vi "StartSeveralKeihtley6221.vi"() -> ()   [LabVIEW 2025]
doc: "Author: Scott Hannahs <sth@magnet.fsu.edu>\n\nThis software is licensed for use under the “MIT License\"\nCopyright (c) 2025 Scott Hannahs, sth@sth@magnet.sthnet.net\n\nPermission is hereby granted, free of charge, to any person obtaining a copy of this software and associated documentation files (the \"Software\"), to deal in the Software without restriction, including without limitation the rights to use, copy, modify, merge, publish, distribute, sublicense, and/or sell copies of the Software, and to permit persons to whom the Software is furnished to do so, subject to the following conditions: The above copyright notice and this permission notice shall be included in all copies or substantial portions of the Software.\n\nTHE SOFTWARE IS PROVIDED \"AS IS\", WITHOUT WARRANTY OF ANY KIND, EXPRESS OR IMPLIED, INCLUDING BUT NOT LIMITED TO THE WARRANTIES OF MERCHANTABILITY, FITNESS FOR A PARTICULAR PURPOSE AND NONINFRINGEMENT. IN NO EVENT SHALL THE AUTHORS OR COPYRIGHT HOLDERS BE LIABLE FOR ANY CLAIM, DAMAGES OR OTHER LIABILITY, WHETHER IN AN ACTION OF CONTRACT, TORT OR OTHERWISE, ARISING FROM, OUT OF OR IN CONNECTION WITH THE SOFTWARE OR THE USE OR OTHER DEALINGS IN THE SOFTWARE."
panel:
  in  "stop":bool
  in  "RUN Button":bool
  in  "MODE":T1(tab)=enum."DELTA mode"
  in  "DELTA HIGH \n(0 --- +0.105 Amp)":dbl=5e-08 min=0.0 max=0.00105 format="%^.5e"
  in  "DELTA LOW \n(-0.105 --- 0 Amp)":dbl=-5e-08 min=-0.00105 max=0.0 format="%^.5e"
  in  "DELTA DELAY \n(0 --- 9999.999 sec)":dbl=0.1 min=0.0 max=9999.999 format="%^.5e"
  in  "Ilow = -Ihigh":bool=TRUE
  in  "Delay of 6221#d \nwith respect to 6221#s\n(sec)":dbl=0.01 min=0.0 max=9999.999 format="%^.5e"
  in  "apperture of 2181A#s \n(NPLC, integer 1 - 60)":dbl=1.0 min=0.0 max=9999.999 format="%^.5e"
  in  "Delay of 2182#d \nwith respect to 2182#s\n(NPLC, integer 1-59)\nType Zero, if serial connection":dbl min=0.0 max=9999.999 format="%^.5e"
  in  "DELAY \n(0 --- 9999.999 sec)":dbl=0.1 min=0.0 max=9999.999 format="%^.5e"
  in  "Time Delay of 6221#d \nwith respect to 6221#s \n(sec)":dbl=0.01 min=0.0 max=9999.999 format="%^.5e"
  in  "Apperture of 2182#s \n(NPLC, integer 1 - 60)":dbl=1.0 min=0.0 max=9999.999 format="%^.5e"
  in  "Delay of 2182#d \nwith respect to 2182#s\n(NPLC, integer 1-59)\nType Zero, if serial connection":dbl=1.0 min=0.0 max=9999.999 format="%^.5e"
  in  "DELTA == dI\n(0 --- +105 mA)":dbl=1e-08 min=0.0 max=0.00105 format="%^.5e"
  in  "STEP \n(0 --- +0.105 Amp)":dbl=2e-09 min=0.0 max=0.00105 format="%^.5e"
  in  "STOP \n(-105 -- +105 mA)":dbl=1e-06 min=-0.001 max=0.00105 format="%^.5e"
  in  "START\n(-105 -- +0.105 mA)":dbl=-1.2e-06 min=-0.001 max=0.00105 format="%^.5e"
  in  "Disable Displays":bool
  in  "Subordinate 6221s: Reinitialize to Default Value \nto reduce the amount of the elements":refnum<visa-resource-name>[](array[refnum])=["GPIB0::17::INSTR"]
  in  "Dominate Current source: 6221#d":refnum<visa-resource-name>="GPIB0::16::INSTR"
  # "Abort Sweep, Delta, Pulse Delta, or Differential Conductance immediately"
  # "Trigger armed mode. For example, Diff. conductance"
  # "1NPLC = 16.6[6]msec"
  # "1NPLC = 16.6[6]msec"
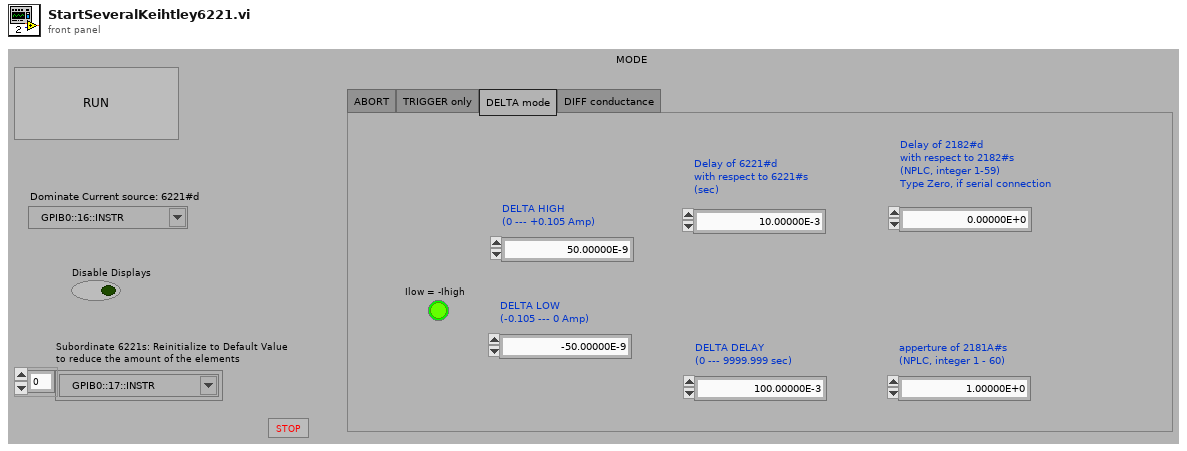
[diagram p1: front panel]
types:
  T1 = enum32{"ABORT", "TRIGGER only", "DELTA mode", "DIFF conductance"}
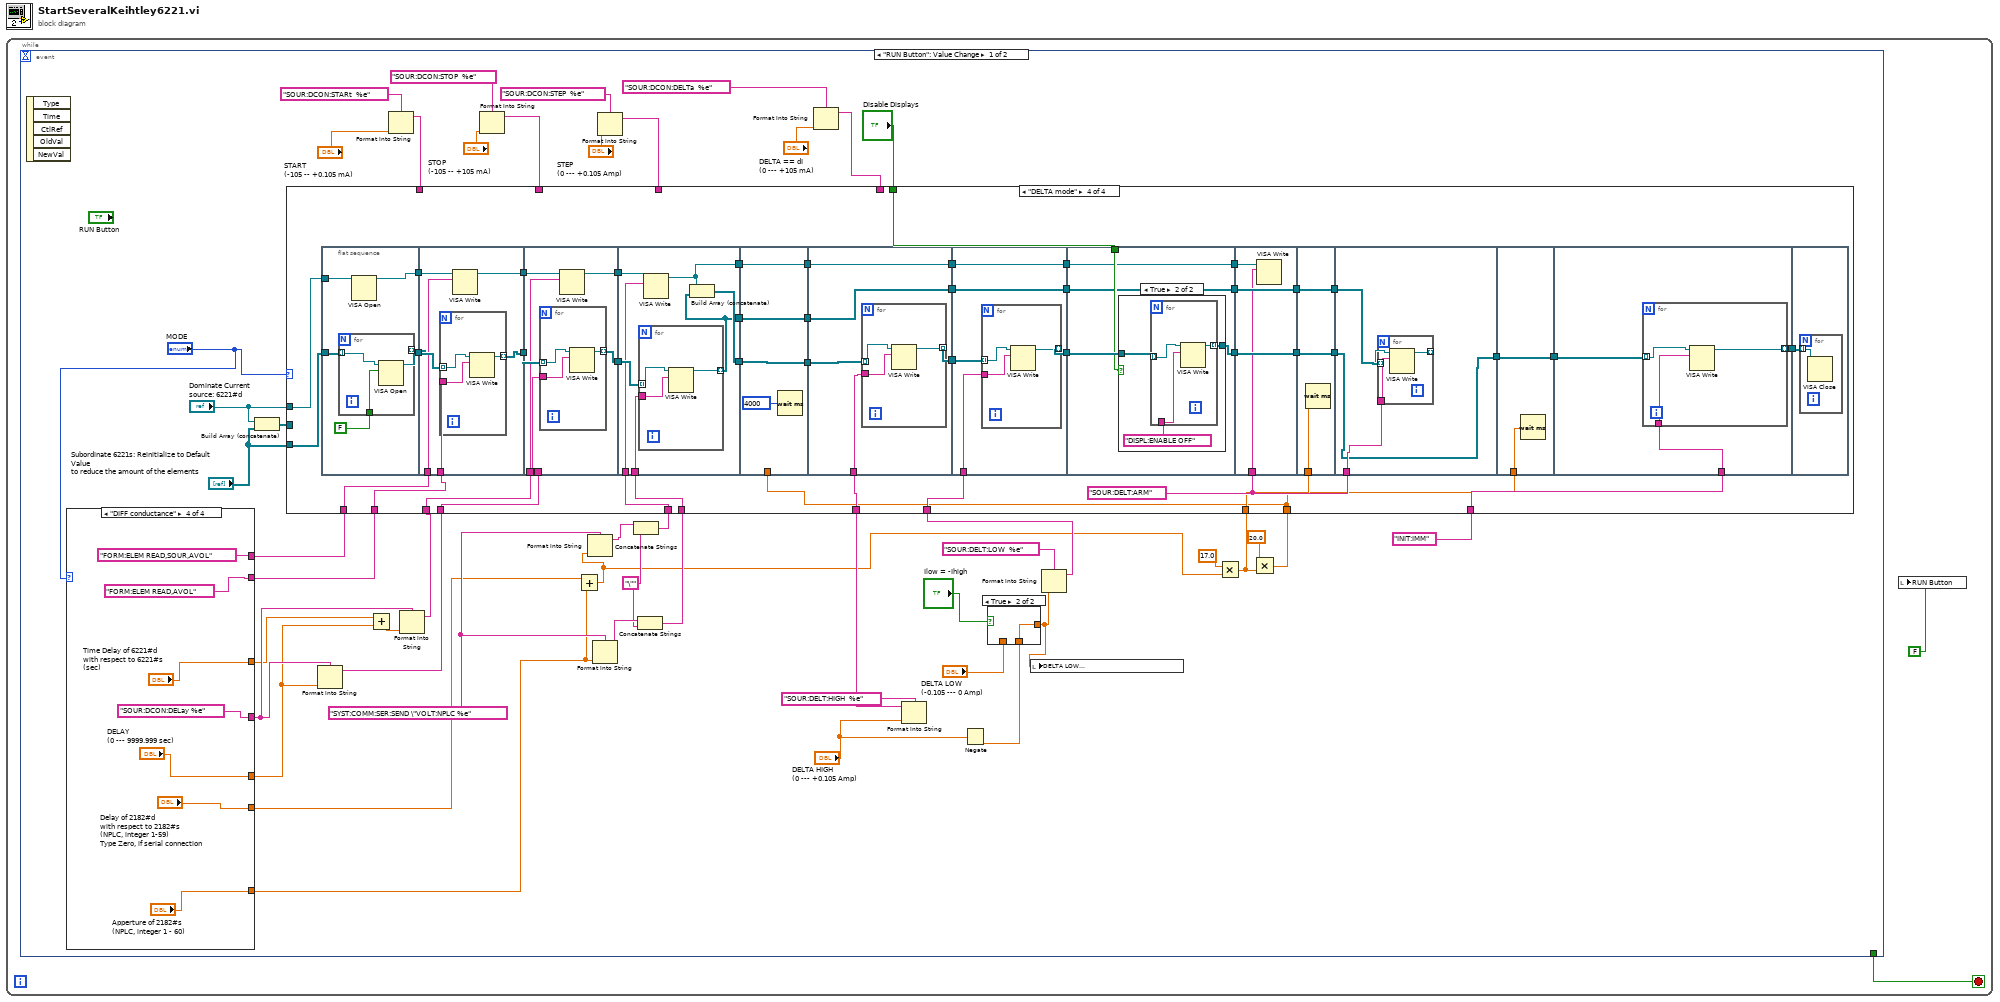
[diagram p0: block diagram]
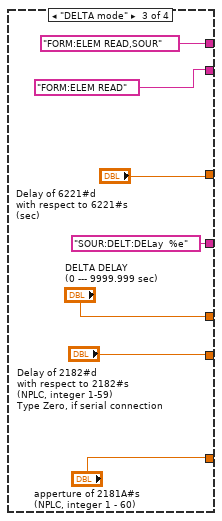
[diagram p4: hidden frame]
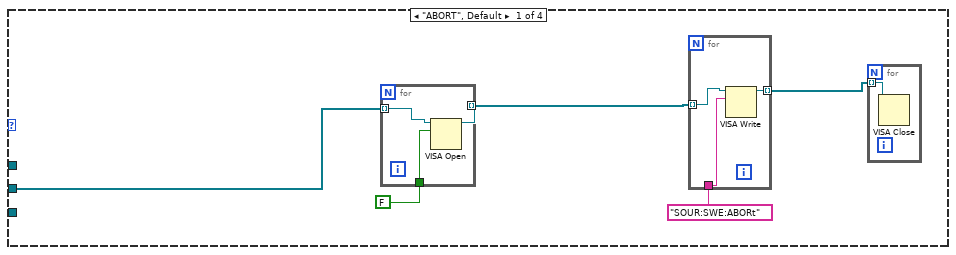
[diagram p5: hidden frame]
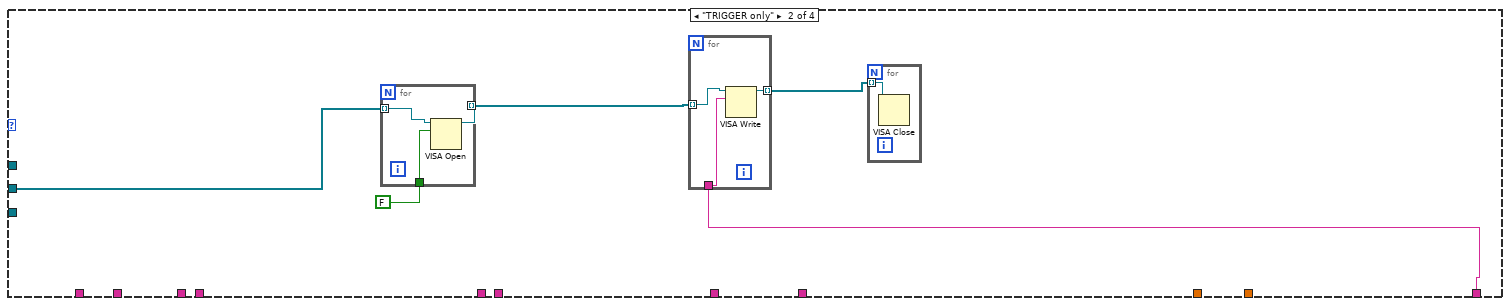
[diagram p6: hidden frame]
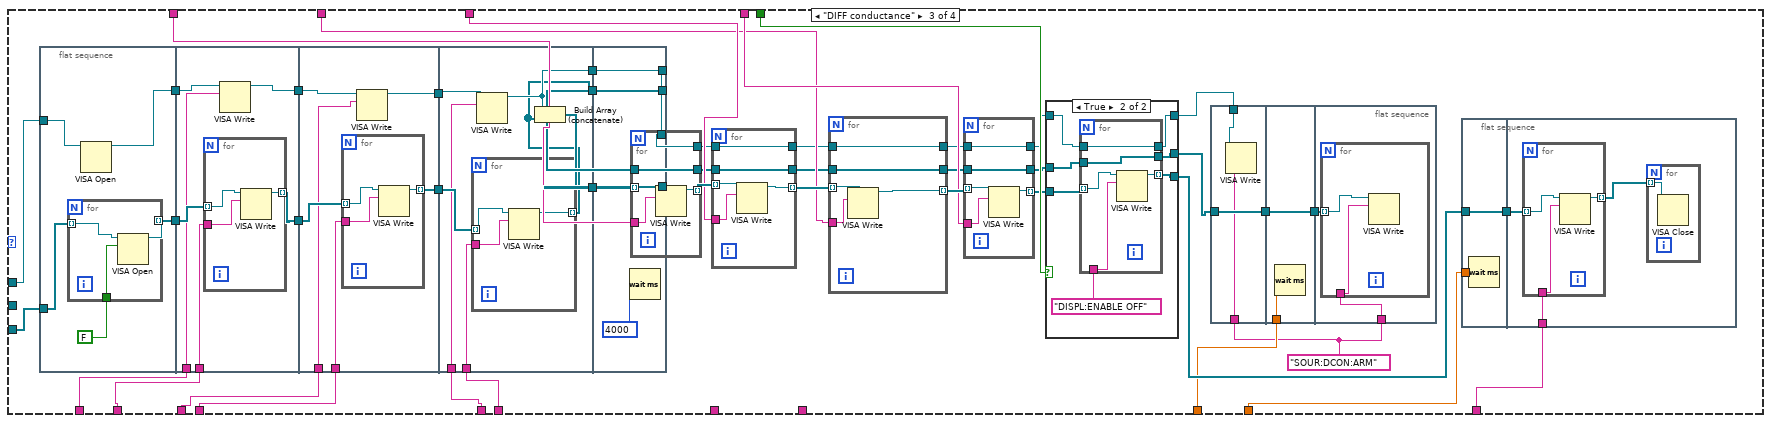
[diagram p7: hidden frame]
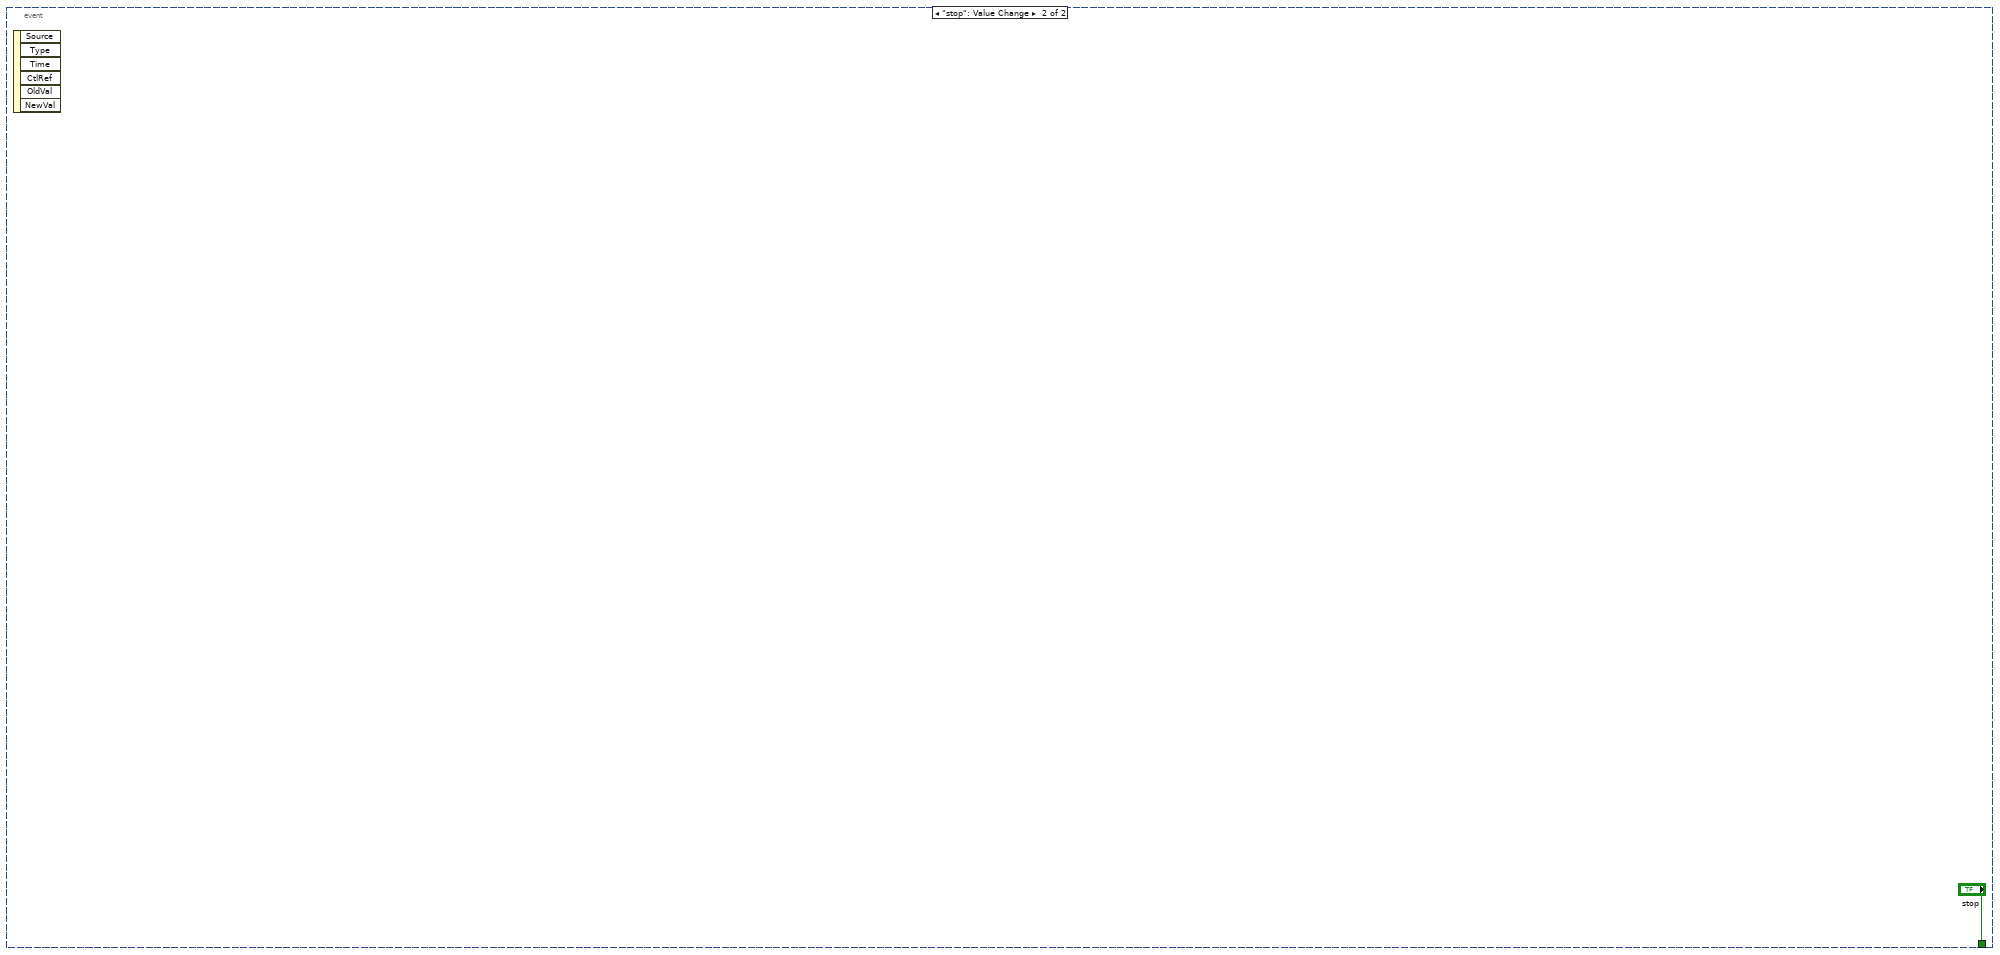
[diagram p11: hidden frame]
diagram:
  n1 = while {
    stop <- w2 stop-if-true
    n2 = event shown="[0] \"RUN Button\": Value Change" {
      selector: _ -> [_ _]
      dyn-events: _ -> [_ _]
      timeout: _ -> [_ _]
      tunnel: [_ "stop"] -> w2
      event "RUN Button": Value Change {
        w31 = "\""
        w34 = "SYST:COMM:SER:SEND \"VOLT:NPLC %e"
        n3 = event-data() -> ()  [unwired: 1 in, 5 out]
        n4 = case shown="\"DIFF conductance\"" "MODE" {
          tunnel: [_ _ "SOUR:DELT:DELay  %e" "SOUR:DCON:DELay %e"] -> w14
          tunnel: [_ _ "DELTA DELAY \n(0 --- 9999.999 sec)" "DELAY \n(0 --- 9999.999 sec)"] -> w13
          tunnel: [_ _ "Delay of 6221#d \nwith respect to 6221#s\n(sec)" "Time Delay of 6221#d \nwith respect to 6221#s \n(sec)"] -> w12
          tunnel: [_ _ "Delay of 2182#d \nwith respect to 2182#s\n(NPLC, integer 1-59)\nType Zero, if serial connection" "Delay of 2182#d \nwith respect to 2182#s\n(NPLC, integer 1-59)\nType Zero, if serial connection"] -> w6
          tunnel: [_ _ "apperture of 2181A#s \n(NPLC, integer 1 - 60)" "Apperture of 2182#s \n(NPLC, integer 1 - 60)"] -> w5
          tunnel: [_ _ "FORM:ELEM READ,SOUR" "FORM:ELEM READ,SOUR,AVOL"] -> w4
          tunnel: [_ _ "FORM:ELEM READ" "FORM:ELEM READ,AVOL"] -> w3
          frame "ABORT", Default {
          }
          frame "TRIGGER only" {
          }
          frame "DELTA mode" {
          }
          frame "DIFF conductance" {
          }
        }
        n5 = Build Array (concatenate)("Dominate Current source: 6221#d", "Subordinate 6221s: Reinitialize to Default Value \nto reduce the amount of the elements") -> (w45:refnum<visa-resource-name>[])
        n6 = Format Into String(format string=w14, w13) -> (resulting string=w48:string)  [unwired: 2 in, 1 out]
        n7 = Add(x=w12, y=w13) -> (x+y=w36:dbl)
        n8 = Format Into String(format string="SOUR:DCON:STARt  %e", "START\n(-105 -- +0.105 mA)") -> (resulting string=w21:string)  [unwired: 2 in, 1 out]
        n9 = Format Into String(format string=w14, w36) -> (resulting string=w35:string)  [unwired: 2 in, 1 out]
        n10 = Format Into String(format string="SOUR:DCON:STOP  %e", "STOP \n(-105 -- +105 mA)") -> (resulting string=w20:string)  [unwired: 2 in, 1 out]
        n11 = Add(x=w6, y=w5) -> (x+y=w10:dbl)
        n12 = Format Into String(format string=w34, w10) -> (resulting string=w33:string)  [unwired: 2 in, 1 out]
        n13 = Format Into String(format string=w34, w5) -> (resulting string=w32:string)  [unwired: 2 in, 1 out]
        n14 = Format Into String(format string="SOUR:DCON:STEP  %e", "STEP \n(0 --- +0.105 Amp)") -> (resulting string=w19:string)  [unwired: 2 in, 1 out]
        n15 = Concatenate Strings(w33, w31) -> (w30:string)
        n16 = Concatenate Strings(w32, w31) -> (w29:string)
        n17 = Format Into String(format string="SOUR:DCON:DELTa  %e", "DELTA == dI\n(0 --- +105 mA)") -> (resulting string=w16:string)  [unwired: 2 in, 1 out]
        n18 = Format Into String(format string="SOUR:DELT:HIGH  %e", "DELTA HIGH \n(0 --- +0.105 Amp)") -> (resulting string=w46:string)  [unwired: 2 in, 1 out]
        n19 = Negate(x="DELTA HIGH \n(0 --- +0.105 Amp)") -> (-x=w40:dbl)
        n20 = case shown="True" "Ilow = -Ihigh" {
          tunnel: "DELTA LOW \n(-0.105 --- 0 Amp)" -> [w363 _]
          tunnel: [w363 w364] -> w42
          tunnel: w40 -> [_ w364]
          frame False {
          }
          frame True {
          }
        }
        n21 = local write "DELTA LOW \n(-0.105 --- 0 Amp)"(w42) -> ()
        n22 = Format Into String(format string="SOUR:DELT:LOW  %e", w42) -> (resulting string=w47:string)  [unwired: 2 in, 1 out]
        n23 = Multiply(x=17.0, y=w10) -> (x*y=w9:dbl)
        n24 = Multiply(x=20.0, y=w9) -> (x*y=w8:dbl)
        n25 = case shown="\"DELTA mode\"" "MODE" {
          tunnel: w48 -> [_ _ w131 w263]
          tunnel: w47 -> [_ _ _ w266]
          tunnel: w46 -> [_ _ _ w265]
          tunnel: w45 -> [w67 w80 _ _]
          tunnel: "Disable Displays" -> [_ _ w135 w268]
          tunnel: "Subordinate 6221s: Reinitialize to Default Value \nto reduce the amount of the elements" -> [_ _ w134 w267]
          tunnel: "Dominate Current source: 6221#d" -> [_ _ w133 w261]
          tunnel: w35 -> [_ _ w132 w262]
          tunnel: w30 -> [_ _ w127 w259]
          tunnel: w29 -> [_ _ w128 w258]
          tunnel: "INIT:IMM" -> [_ w77 w120 w257]
          tunnel: w21 -> [_ _ w125 _]
          tunnel: w20 -> [_ _ w107 _]
          tunnel: w19 -> [_ _ w108 _]
          tunnel: w16 -> [_ _ w121 _]
          tunnel: w8 -> [_ _ w117 w235]
          tunnel: w9 -> [_ _ w113 w242]
          tunnel: w4 -> [_ _ w90 w230]
          tunnel: w3 -> [_ _ w89 w229]
          frame "ABORT", Default {
            n26 = for {
              tunnel: w67 -> [w72] mode=indexing
              tunnel: [w71] -> w66 mode=indexing
              tunnel: FALSE ("duplicate session (F)") -> [w70]
              n27 = VISA Open(duplicate session (F)=w70, VISA resource name=w72) -> (VISA resource name=w71:refnum<visa-resource-name>)  [unwired: 3 in, 1 out]
            }
            n28 = for {
              tunnel: w66 -> [w74] mode=indexing
              tunnel: "SOUR:SWE:ABORt" ("String to Write") -> [w75]
              tunnel: [w73] -> w65 mode=indexing
              n29 = VISA Write(VISA resource name=w74, write buffer=w75) -> (VISA resource name out=w73:refnum<visa-resource-name>)  [unwired: 1 in, 2 out]
            }
            n30 = for {
              tunnel: w65 -> [w76] mode=indexing
              n31 = VISA Close(VISA resource name=w76) -> ()  [unwired: 1 in, 1 out]
            }
          }
          frame "TRIGGER only" {
            n32 = for {
              tunnel: w80 -> [w84] mode=indexing
              tunnel: [w83] -> w79 mode=indexing
              tunnel: FALSE ("duplicate session (F)") -> [w82]
              n33 = VISA Open(duplicate session (F)=w82, VISA resource name=w84) -> (VISA resource name=w83:refnum<visa-resource-name>)  [unwired: 3 in, 1 out]
            }
            n34 = for {
              tunnel: w79 -> [w86] mode=indexing
              tunnel: w77 -> [w87]
              tunnel: [w85] -> w78 mode=indexing
              n35 = VISA Write(VISA resource name=w86, write buffer=w87) -> (VISA resource name out=w85:refnum<visa-resource-name>)  [unwired: 1 in, 2 out]
            }
            n36 = for {
              tunnel: w78 -> [w88] mode=indexing
              n37 = VISA Close(VISA resource name=w88) -> ()  [unwired: 1 in, 1 out]
            }
          }
          frame "DIFF conductance" {
            w112 = "SOUR:DCON:ARM" ("String to Write")
            n38 = flat-sequence {
              tunnel: w134 -> [w178]
              tunnel: w133 -> [w176]
              tunnel: [w177] -> w94
              tunnel: [w174] -> w92
              tunnel: w94 -> [w186]
              tunnel: [w187] -> w93
              tunnel: w92 -> [w184]
              tunnel: [w185] -> w91
              tunnel: w90 -> [w183]
              tunnel: w89 -> [w182]
              tunnel: w93 -> [w196]
              tunnel: w91 -> [w195]
              tunnel: w132 -> [w194]
              tunnel: w131 -> [w193]
              tunnel: [w192] -> w130
              tunnel: [w191] -> w129
              tunnel: w130 -> [w206]
              tunnel: w129 -> [w205]
              tunnel: w127 -> [w204]
              tunnel: w128 -> [w203]
              tunnel: [w202] -> w111
              tunnel: [w201] -> w110
              tunnel: [w200] -> w109
              tunnel: [w211] -> w106
              tunnel: [w212] -> w100
              tunnel: [w213] -> w126
              tunnel: w111 -> [w213]
              tunnel: w110 -> [w212]
              tunnel: w109 -> [w211]
              frame #0 {
                n39 = for {
                  tunnel: w178 -> [w181] mode=indexing
                  tunnel: [w180] -> w177 mode=indexing
                  tunnel: FALSE ("duplicate session (F)") -> [w179]
                  n40 = VISA Open(duplicate session (F)=w179, VISA resource name=w181) -> (VISA resource name=w180:refnum<visa-resource-name>)  [unwired: 3 in, 1 out]
                }
                n41 = VISA Open(VISA resource name=w176) -> (VISA resource name=w174:refnum<visa-resource-name>)  [unwired: 4 in, 1 out]
              }
              frame #1 {
                n42 = for {
                  tunnel: w186 -> [w189] mode=indexing
                  tunnel: w182 -> [w190]
                  tunnel: [w188] -> w187 mode=indexing
                  n43 = VISA Write(VISA resource name=w189, write buffer=w190) -> (VISA resource name out=w188:refnum<visa-resource-name>)  [unwired: 1 in, 2 out]
                }
                n44 = VISA Write(VISA resource name=w184, write buffer=w183) -> (VISA resource name out=w185:refnum<visa-resource-name>)  [unwired: 1 in, 2 out]
              }
              frame #2 {
                n45 = for {
                  tunnel: w196 -> [w198] mode=indexing
                  tunnel: w193 -> [w199]
                  tunnel: [w197] -> w191 mode=indexing
                  n46 = VISA Write(VISA resource name=w198, write buffer=w199) -> (VISA resource name out=w197:refnum<visa-resource-name>)  [unwired: 1 in, 2 out]
                }
                n47 = VISA Write(VISA resource name=w195, write buffer=w194) -> (VISA resource name out=w192:refnum<visa-resource-name>)  [unwired: 1 in, 2 out]
              }
              frame #3 {
                n48 = for {
                  tunnel: w203 -> [w209]
                  tunnel: [w208] -> w200 mode=indexing
                  tunnel: w205 -> [w207] mode=indexing
                  n49 = VISA Write(VISA resource name=w207, write buffer=w209) -> (VISA resource name out=w208:refnum<visa-resource-name>)  [unwired: 1 in, 2 out]
                }
                n50 = VISA Write(VISA resource name=w206, write buffer=w204) -> (VISA resource name out=w201:refnum<visa-resource-name>)  [unwired: 1 in, 2 out]
                n51 = Build Array (concatenate)(w201, w200) -> (w202:refnum<visa-resource-name>[])
              }
              frame #4 {
                n52 = Wait (ms)(milliseconds to wait=u32 4000) -> ()  [unwired: 1 out]
              }
            }
            n53 = for {
              tunnel: w125 -> [w173]
              tunnel: [w172] -> w123 mode=indexing
              tunnel: w126 -> [w171] mode=indexing
              tunnel: w106 -> [w170]
              tunnel: [w170] -> w105
              tunnel: w100 -> [w169]
              tunnel: [w169] -> w99
              n54 = VISA Write(VISA resource name=w171, write buffer=w173) -> (VISA resource name out=w172:refnum<visa-resource-name>)  [unwired: 1 in, 2 out]
            }
            n55 = for {
              tunnel: w108 -> [w168]
              tunnel: [w167] -> w124 mode=indexing
              tunnel: w123 -> [w166] mode=indexing
              tunnel: w105 -> [w165]
              tunnel: [w165] -> w104
              tunnel: w99 -> [w164]
              tunnel: [w164] -> w98
              n56 = VISA Write(VISA resource name=w166, write buffer=w168) -> (VISA resource name out=w167:refnum<visa-resource-name>)  [unwired: 1 in, 2 out]
            }
            n57 = for {
              tunnel: w107 -> [w140]
              tunnel: [w139] -> w122 mode=indexing
              tunnel: w124 -> [w138] mode=indexing
              tunnel: w104 -> [w137]
              tunnel: [w137] -> w103
              tunnel: w98 -> [w136]
              tunnel: [w136] -> w97
              n58 = VISA Write(VISA resource name=w138, write buffer=w140) -> (VISA resource name out=w139:refnum<visa-resource-name>)  [unwired: 1 in, 2 out]
            }
            n59 = for {
              tunnel: w121 -> [w163]
              tunnel: [w162] -> w119 mode=indexing
              tunnel: w122 -> [w161] mode=indexing
              tunnel: w103 -> [w160]
              tunnel: [w160] -> w102
              tunnel: w97 -> [w159]
              tunnel: [w159] -> w96
              n60 = VISA Write(VISA resource name=w161, write buffer=w163) -> (VISA resource name out=w162:refnum<visa-resource-name>)  [unwired: 1 in, 2 out]
            }
            n61 = case shown="True" w135 {
              tunnel: w119 -> [w216 w222]
              tunnel: [w216 w221] -> w114
              tunnel: w102 -> [w215 w220]
              tunnel: [w215 w219] -> w101
              tunnel: w96 -> [w214 w218]
              tunnel: [w214 w217] -> w95
              frame False {
              }
              frame True {
                n62 = for {
                  tunnel: w222 -> [w227] mode=indexing
                  tunnel: "DISPL:ENABLE OFF" ("String to Write") -> [w228]
                  tunnel: [w226] -> w221 mode=indexing
                  tunnel: w220 -> [w225]
                  tunnel: [w225] -> w219
                  tunnel: w218 -> [w224]
                  tunnel: [w224] -> w217
                  n63 = VISA Write(VISA resource name=w227, write buffer=w228) -> (VISA resource name out=w226:refnum<visa-resource-name>)  [unwired: 1 in, 2 out]
                }
              }
            }
            n64 = flat-sequence {
              tunnel: w101 -> [w143]
              tunnel: [w143] -> w115
              tunnel: w112 -> [w142]
              tunnel: w95 -> [w141]
              tunnel: [w145] -> w116
              tunnel: w115 -> [w145]
              tunnel: w113 -> [w144]
              tunnel: w112 -> [w146]
              tunnel: w116 -> [w147]
              frame #0 {
                n65 = VISA Write(VISA resource name=w141, write buffer=w142) -> ()  [unwired: 1 in, 3 out]
              }
              frame #1 {
                n66 = Wait (ms)(milliseconds to wait=w144) -> ()  [unwired: 1 out]
              }
              frame #2 {
                n67 = for {
                  tunnel: w147 -> [w148] mode=indexing
                  tunnel: w146 -> [w149]
                  n68 = VISA Write(VISA resource name=w148, write buffer=w149) -> ()  [unwired: 1 in, 3 out]
                }
              }
            }
            n69 = flat-sequence {
              tunnel: w114 -> [w151]
              tunnel: [w151] -> w118
              tunnel: w117 -> [w150]
              tunnel: w120 -> [w152]
              tunnel: w118 -> [w153]
              frame #0 {
                n70 = Wait (ms)(milliseconds to wait=w150) -> ()  [unwired: 1 out]
              }
              frame #1 {
                n71 = for {
                  tunnel: w153 -> [w156] mode=indexing
                  tunnel: w152 -> [w157]
                  tunnel: [w155] -> w154 mode=indexing
                  n72 = VISA Write(VISA resource name=w156, write buffer=w157) -> (VISA resource name out=w155:refnum<visa-resource-name>)  [unwired: 1 in, 2 out]
                }
                n73 = for {
                  tunnel: w154 -> [w158] mode=indexing
                  n74 = VISA Close(VISA resource name=w158) -> ()  [unwired: 1 in, 1 out]
                }
              }
            }
          }
          frame "DELTA mode" {
            w250 = "SOUR:DELT:ARM" ("String to Write")
            n75 = flat-sequence {
              tunnel: w267 -> [w276]
              tunnel: [w275] -> w234
              tunnel: [w273] -> w232
              tunnel: w261 -> [w272]
              tunnel: w234 -> [w282]
              tunnel: [w285] -> w233
              tunnel: w232 -> [w283]
              tunnel: [w284] -> w231
              tunnel: w230 -> [w281]
              tunnel: w229 -> [w280]
              tunnel: w233 -> [w294]
              tunnel: [w293] -> w264
              tunnel: w263 -> [w292]
              tunnel: w262 -> [w291]
              tunnel: w231 -> [w290]
              tunnel: [w289] -> w260
              tunnel: w264 -> [w303]
              tunnel: [w300] -> w241
              tunnel: w260 -> [w304]
              tunnel: w259 -> [w302]
              tunnel: w258 -> [w301]
              tunnel: [w299] -> w239
              tunnel: [w298] -> w237
              tunnel: w241 -> [w311]
              tunnel: [w311] -> w240
              tunnel: w239 -> [w310]
              tunnel: [w310] -> w238
              tunnel: w237 -> [w309]
              tunnel: [w309] -> w236
              tunnel: w235 -> [_]
              tunnel: w240 -> [w316]
              tunnel: [w315] -> w271
              tunnel: w265 -> [w314]
              tunnel: w238 -> [w313]
              tunnel: [w313] -> w253
              tunnel: w236 -> [w312]
              tunnel: [w312] -> w247
              tunnel: [w323] -> w270
              tunnel: w271 -> [w324]
              tunnel: w266 -> [w322]
              tunnel: [w321] -> w254
              tunnel: w253 -> [w321]
              tunnel: [w320] -> w248
              tunnel: w247 -> [w320]
              tunnel: w270 -> [w332]
              tunnel: [w331] -> w252
              tunnel: w268 -> [w330]
              tunnel: [w329] -> w251
              tunnel: w254 -> [w329]
              tunnel: [w328] -> w249
              tunnel: w248 -> [w328]
              tunnel: w252 -> [w343]
              tunnel: [w343] -> w246
              tunnel: w251 -> [w342]
              tunnel: [w342] -> w244
              tunnel: w250 -> [w341]
              tunnel: w249 -> [w340]
              tunnel: w246 -> [w346]
              tunnel: [w346] -> w245
              tunnel: w244 -> [w345]
              tunnel: [w345] -> w243
              tunnel: w242 -> [w344]
              tunnel: [w348] -> w256
              tunnel: w245 -> [w348]
              tunnel: w250 -> [w349]
              tunnel: w243 -> [w347]
              tunnel: w256 -> [w354]
              tunnel: [w354] -> w255
              tunnel: w235 -> [w353]
              tunnel: w255 -> [w357]
              tunnel: [w356] -> w269
              tunnel: w257 -> [w355]
              tunnel: w269 -> [w361]
              frame #0 {
                n76 = for {
                  tunnel: w276 -> [w279] mode=indexing
                  tunnel: [w278] -> w275 mode=indexing
                  tunnel: FALSE ("duplicate session (F)") -> [w277]
                  n77 = VISA Open(duplicate session (F)=w277, VISA resource name=w279) -> (VISA resource name=w278:refnum<visa-resource-name>)  [unwired: 3 in, 1 out]
                }
                n78 = VISA Open(VISA resource name=w272) -> (VISA resource name=w273:refnum<visa-resource-name>)  [unwired: 4 in, 1 out]
              }
              frame #1 {
                n79 = for {
                  tunnel: w282 -> [w287] mode=indexing
                  tunnel: w280 -> [w288]
                  tunnel: [w286] -> w285 mode=indexing
                  n80 = VISA Write(VISA resource name=w287, write buffer=w288) -> (VISA resource name out=w286:refnum<visa-resource-name>)  [unwired: 1 in, 2 out]
                }
                n81 = VISA Write(VISA resource name=w283, write buffer=w281) -> (VISA resource name out=w284:refnum<visa-resource-name>)  [unwired: 1 in, 2 out]
              }
              frame #2 {
                n82 = for {
                  tunnel: w294 -> [w296] mode=indexing
                  tunnel: w292 -> [w297]
                  tunnel: [w295] -> w293 mode=indexing
                  n83 = VISA Write(VISA resource name=w296, write buffer=w297) -> (VISA resource name out=w295:refnum<visa-resource-name>)  [unwired: 1 in, 2 out]
                }
                n84 = VISA Write(VISA resource name=w290, write buffer=w291) -> (VISA resource name out=w289:refnum<visa-resource-name>)  [unwired: 1 in, 2 out]
              }
              frame #3 {
                n85 = for {
                  tunnel: w301 -> [w307]
                  tunnel: [w306] -> w299 mode=indexing
                  tunnel: w303 -> [w305] mode=indexing
                  n86 = VISA Write(VISA resource name=w305, write buffer=w307) -> (VISA resource name out=w306:refnum<visa-resource-name>)  [unwired: 1 in, 2 out]
                }
                n87 = VISA Write(VISA resource name=w304, write buffer=w302) -> (VISA resource name out=w298:refnum<visa-resource-name>)  [unwired: 1 in, 2 out]
                n88 = Build Array (concatenate)(w298, w299) -> (w300:refnum<visa-resource-name>[])
              }
              frame #4 {
                n89 = Wait (ms)(milliseconds to wait=u32 4000) -> ()  [unwired: 1 out]
              }
              frame #5 {
                n90 = for {
                  tunnel: w314 -> [w319]
                  tunnel: [w318] -> w315 mode=indexing
                  tunnel: w316 -> [w317] mode=indexing
                  n91 = VISA Write(VISA resource name=w317, write buffer=w319) -> (VISA resource name out=w318:refnum<visa-resource-name>)  [unwired: 1 in, 2 out]
                }
              }
              frame #6 {
                n92 = for {
                  tunnel: w324 -> [w326] mode=indexing
                  tunnel: w322 -> [w327]
                  tunnel: [w325] -> w323 mode=indexing
                  n93 = VISA Write(VISA resource name=w326, write buffer=w327) -> (VISA resource name out=w325:refnum<visa-resource-name>)  [unwired: 1 in, 2 out]
                }
              }
              frame #7 {
                n94 = case shown="True" w330 {
                  tunnel: w332 -> [w333 w335]
                  tunnel: [w333 w334] -> w331
                  frame False {
                  }
                  frame True {
                    n95 = for {
                      tunnel: w335 -> [w338] mode=indexing
                      tunnel: "DISPL:ENABLE OFF" ("String to Write") -> [w339]
                      tunnel: [w337] -> w334 mode=indexing
                      n96 = VISA Write(VISA resource name=w338, write buffer=w339) -> (VISA resource name out=w337:refnum<visa-resource-name>)  [unwired: 1 in, 2 out]
                    }
                  }
                }
              }
              frame #8 {
                n97 = VISA Write(VISA resource name=w340, write buffer=w341) -> ()  [unwired: 1 in, 3 out]
              }
              frame #9 {
                n98 = Wait (ms)(milliseconds to wait=w344) -> ()  [unwired: 1 out]
              }
              frame #10 {
                n99 = for {
                  tunnel: w347 -> [w351] mode=indexing
                  tunnel: w349 -> [w352]
                  tunnel: [w350] -> _ mode=indexing
                  n100 = VISA Write(VISA resource name=w351, write buffer=w352) -> (VISA resource name out=w350:refnum<visa-resource-name>)  [unwired: 1 in, 2 out]
                }
              }
              frame #11 {
                n101 = Wait (ms)(milliseconds to wait=w353) -> ()  [unwired: 1 out]
              }
              frame #12 {
                n102 = for {
                  tunnel: w355 -> [w360]
                  tunnel: w357 -> [w359] mode=indexing
                  tunnel: [w358] -> w356 mode=indexing
                  n103 = VISA Write(VISA resource name=w359, write buffer=w360) -> (VISA resource name out=w358:refnum<visa-resource-name>)  [unwired: 1 in, 2 out]
                }
              }
              frame #13 {
                n104 = for {
                  tunnel: w361 -> [w362] mode=indexing
                  n105 = VISA Close(VISA resource name=w362) -> ()  [unwired: 1 in, 1 out]
                }
              }
            }
          }
        }
      }
      event "stop": Value Change {
        n106 = event-data() -> ()  [unwired: 1 in, 6 out]
      }
    }
    n107 = local write "RUN Button"(FALSE ("RUN Button")) -> ()
  }
